vi "2d_interpolation.vi"() -> ()   [LabVIEW 2014]
uses:
  <vilib>/Analysis/NI_AALPro.lvlib
panel:
  in  "Interpolation factor":i32=10
  out "Interpolated array":dbl[][](array[numeric]) format="%.2f"
  in  "Input array":dbl[][](array[numeric])
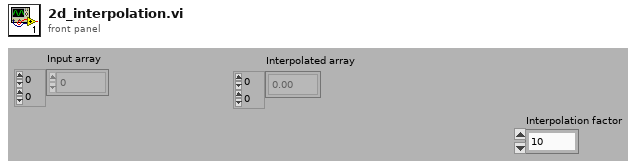
[diagram p1: front panel]
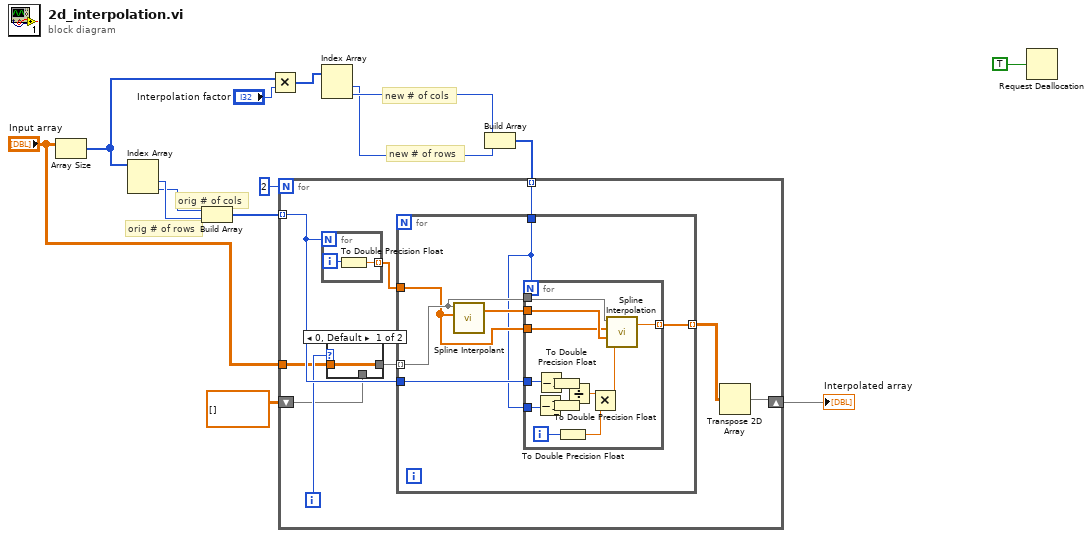
[diagram p0: block diagram]
diagram:
  # "new # of rows"
  # "new # of cols"
  # "orig # of rows"
  # "orig # of cols"
  n1 = Array Size(array="Input array") -> (size(s)=w5:i32[])
  n2 = Index Array(array=w5) -> (element #1=w2:i32, element #2=w1:i32)  [unwired: 2 in]
  n3 = Build Array(w1, w2) -> (w11:i32[])
  n4 = Multiply(x=w5, y="Interpolation factor") -> (x*y=w7:i32[])
  n5 = Index Array(array=w7) -> (element #1=w3:i32, element #2=w4:i32)  [unwired: 2 in]
  n6 = Build Array(w4, w3) -> (w12:i32[])
  n7 = for {
    N: 2 -> [_]
    tunnel: "Input array" -> [w19]
    tunnel: w11 -> [w21] mode=indexing
    shift-right: [w15] -> w8
    shift-left: dbl[][] [] -> [w17]
    tunnel: w12 -> [w16] mode=indexing
    i -> [w20]
    n8 = for {
      N: w21 -> [_]
      tunnel: [w26] -> w23 mode=indexing
      i -> [w27]
      n9 = To Double Precision Float(number=w27) -> (double precision float=w26:dbl)
    }
    n10 = case shown="0, Default" w20 {
      tunnel: w19 -> [w24 _]
      tunnel: [w24 w25] -> w18
      tunnel: w17 -> [_ w25]
      frame 0, Default {
      }
      frame 1 {
      }
    }
    n11 = for {
      tunnel: w21 -> [w33]
      tunnel: w18 -> [w31] mode=indexing
      tunnel: w23 -> [w30]
      tunnel: [w29] -> w22 mode=indexing
      tunnel: w16 -> [w28]
      n12 = call <vilib>:"Spline Interpolant.vi"("X"=w30, "Y"=w31) -> ("Interpolant"=w32:dbl[])  [unwired: 2 in, 1 out]
      n13 = for {
        N: w28 -> [_]
        tunnel: w33 -> [w44]
        tunnel: w32 -> [w42]
        tunnel: w31 -> [w41]
        tunnel: w30 -> [w40]
        tunnel: [w39] -> w29 mode=indexing
        tunnel: w28 -> [w37]
        i -> [w43]
        n14 = Decrement(x=w37) -> (x-1=w46:i32)
        n15 = Decrement(x=w44) -> (x-1=w47:i32)
        n16 = To Double Precision Float(number=w47) -> (double precision float=w35:dbl)
        n17 = To Double Precision Float(number=w46) -> (double precision float=w34:dbl)
        n18 = To Double Precision Float(number=w43) -> (double precision float=w36:dbl)
        n19 = Divide(x=w35, y=w34) -> (x/y=w45:dbl)
        n20 = Multiply(x=w45, y=w36) -> (x*y=w38:dbl)
        n21 = call <vilib>:"Spline Interpolation.vi"("x value"=w38, "Interpolant"=w42, "X"=w40, "Y"=w41) -> ("interpolation value"=w39:dbl)  [unwired: 1 out]
      }
    }
    n22 = Transpose 2D Array(2D array=w22) -> (transposed array=w15:dbl[][])
  }
  "Interpolated array" <- w8
  n23 = Request Deallocation(TRUE ("flag")) -> ()
